vi "SetShieldRef.vi"(8 "error in (no error)":errorcluster, 10 "Motorshield Ref in":refnum<vi>, 11 "DCMotor in":refnum<class "DCMotor.lvclass">) -> (0 "error out":errorcluster, 3 "DCMotor out":refnum<class "DCMotor.lvclass">)   [LabVIEW 2022 SP3, in "Motorshield.lvlib" / "DCMotor.lvclass"]
uses:
  DCMotor.lvclass
  DCMotor.lvclass/DCMotor.ctl
  Motorshield/Motorshield.lvclass
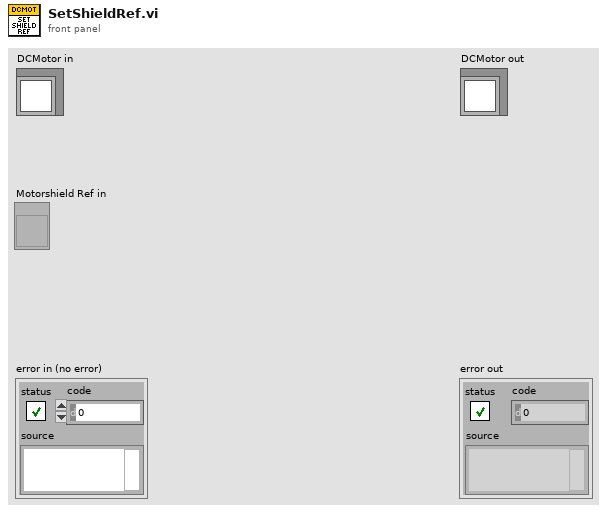
[diagram p1: front panel]
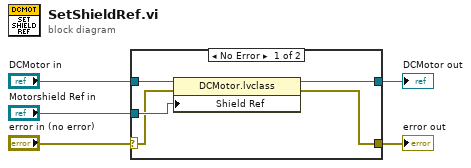
[diagram p0: block diagram]
diagram:
  n1 = case shown="No Error" "error in (no error)" {
    selector: "error in (no error)" -> [w7 w12]
    tunnel: [w6 w12] -> w4
    tunnel: [w9 w11] -> w2
    tunnel: "DCMotor in" -> [w10 w11]
    tunnel: "Motorshield Ref in" -> [w8 _]
    frame No Error {
      n2 = property class="DCMotor.lvclass"(reference=w10, error in=w7, "Shield Ref"=w8) -> (reference out=w9:refnum<class "DCMotor.lvclass">, error out=w6:errorcluster)
    }
    frame Error {
    }
  }
  "error out" <- w4
  "DCMotor out" <- w2
